vi "XBox-Stop Controller.vi"   [LabVIEW 2015]
uses:
  XBox-Globals.vi
panel:
  # "All this does is set a global variable to stop the XBox controller which is presumably running in the background. The purpose is to hide the global variables from the higher-level applications. There is probably a better way to do this sort of thing; whatever that is can be plugged into this VI in the future, without disrupting existing applications."
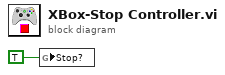
[diagram p0: block diagram]
diagram:
  n1 = global write "XBox-Globals.vi" "Stop?"(TRUE ("Stop?")) -> ()
